vi "ComputeROIArray.vi"(7 "ROIDim":T1, 8 "error in (no error)":errorcluster, 10 "ROI In":T2 {"Contours"."Type" items=["No Selection", "Point", "Line", "Rectangle", "Oval", "Polygon", "Freehand Region", "Annulus", "Unused2", "Unused3", "Broken Line", "Freehand Line", "Rotated Rectangle"]}) -> (0 "error out":errorcluster, 2 "ROIs Out":T2[](array[typedef]) {"Contours"."Type" items=["No Selection", "Point", "Line", "Rectangle", "Oval", "Polygon", "Freehand Region", "Annulus", "Unused2", "Unused3", "Broken Line", "Freehand Line", "Rotated Rectangle"]})   [LabVIEW 2019]
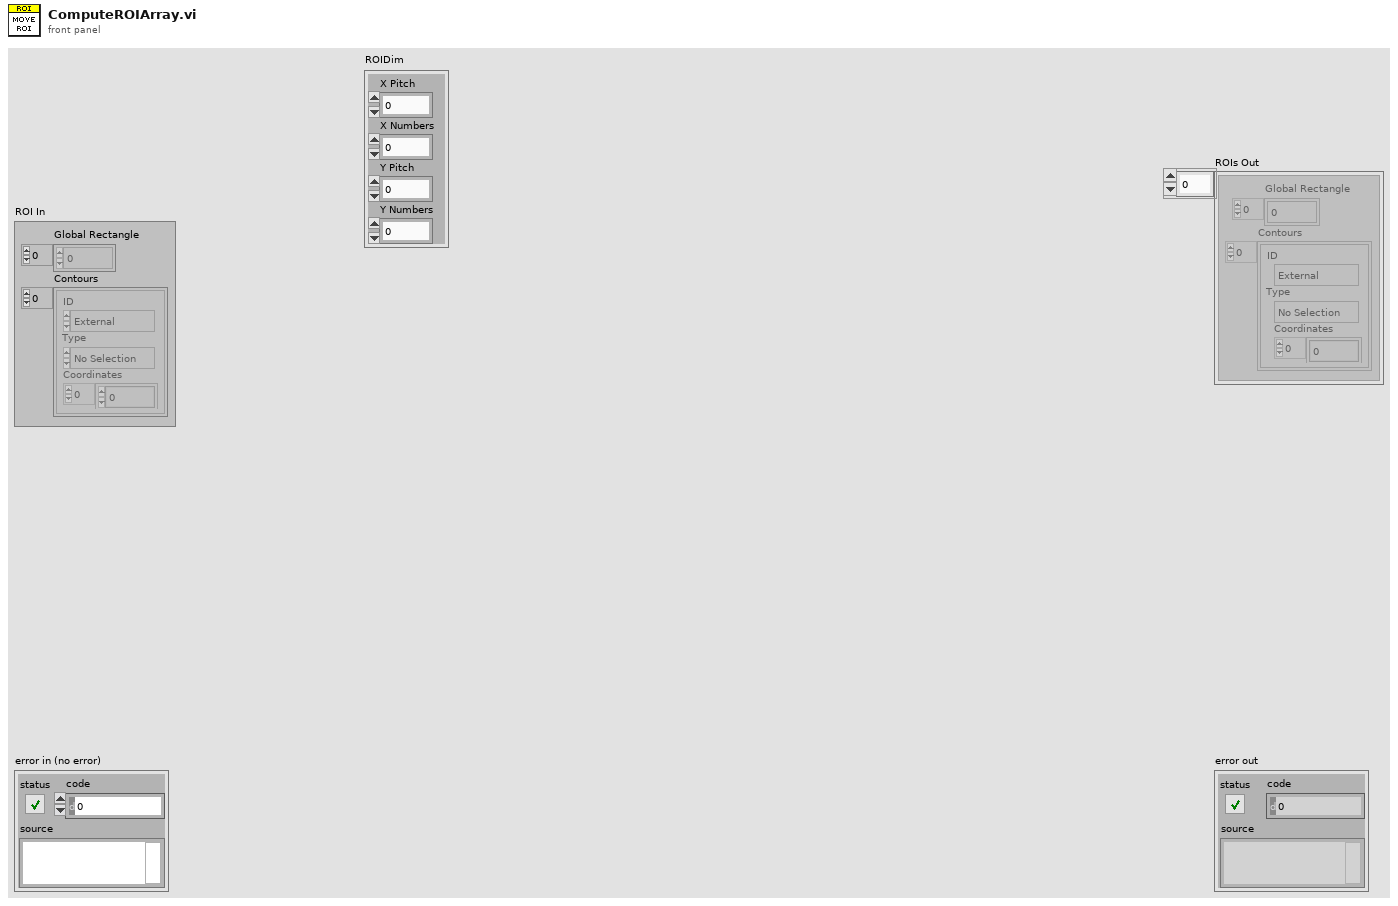
[diagram p1: front panel]
types:
  T1 = cluster{"X Pitch":i32, "X Numbers":i32, "Y Pitch":i32, "Y Numbers":i32}
  T2 = typedef "ROI Descriptor" = cluster{"Global Rectangle":i32[], "Contours":cluster{"ID":enum32{"External", "Internal"}, "Type":u32, "Coordinates":i32[]}[]}
  T3 = cluster{"ID":enum32{"External", "Internal"}, "Type":u32, "Coordinates":i32[]}[]
  T4 = cluster{"ID":enum32{"External", "Internal"}, "Type":u32, "Coordinates":i32[]}
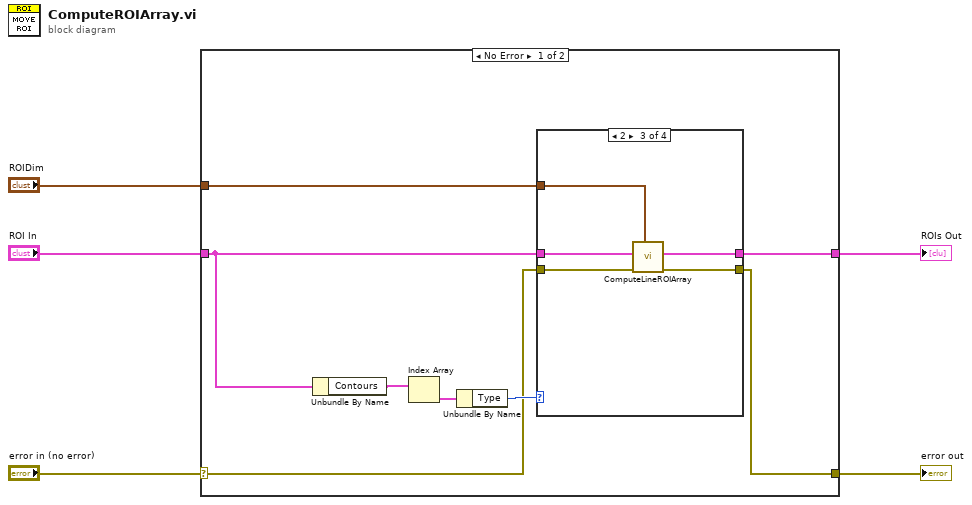
[diagram p0: block diagram]
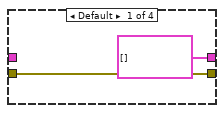
[diagram p2: hidden frame]
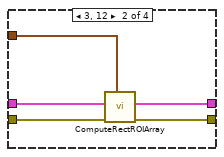
[diagram p3: hidden frame]
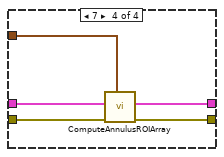
[diagram p4: hidden frame]
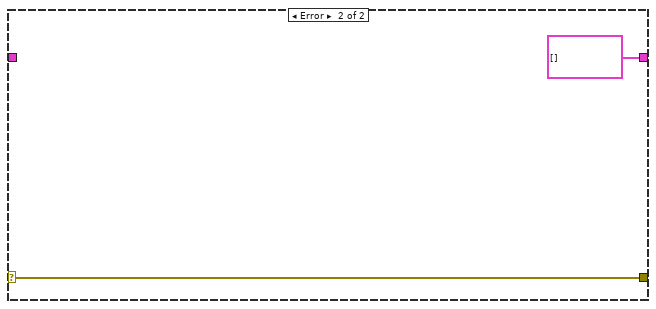
[diagram p5: hidden frame]
diagram:
  n1 = case shown="No Error" "error in (no error)" {
    selector: "error in (no error)" -> [w9 w32]
    tunnel: "ROI In" -> [w13 _]
    tunnel: [w8 w32] -> w3
    tunnel: [w7 T2[] [] ("ROIArray")] -> w2
    tunnel: "ROIDim" -> [w6 _]
    frame No Error {
      n2 = Unbundle By Name(w13) -> ("Contours"=w12:T3)
      n3 = Index Array(array=w12) -> (element=w11:T4)  [unwired: 1 in]
      n4 = Unbundle By Name(w11) -> ("Type"=w10:u32)
      n5 = case shown="2" w10 {
        tunnel: [T2[] [] ("ROIArray") w20 w25 w30] -> w7
        tunnel: [w15 w19 w24 w29] -> w8
        tunnel: w13 -> [_ w18 w22 w28]
        tunnel: w9 -> [w15 w17 w23 w27]
        tunnel: w6 -> [_ w16 w21 w26]
        frame Default {
        }
        frame 3, 12 {
          n6 = call "ComputeRectROIArray.vi"("ROIDim"=w16, "error in (no error)"=w17, "ROI In"=w18) -> ("error out"=w19:errorcluster, "ROIArray"=w20:T2[])  [unwired: 7 in]
        }
        frame 2 {
          n7 = call "ComputeLineROIArray.vi"("ROIDim"=w21, "error in (no error)"=w23, "ROI In"=w22) -> ("error out"=w24:errorcluster, "ROIArray"=w25:T2[])  [unwired: 7 in]
        }
        frame 7 {
          n8 = call "ComputeAnnulusROIArray.vi"("ROIDim"=w26, "error in (no error)"=w27, "ROI In"=w28) -> ("error out"=w29:errorcluster, "ROIArray"=w30:T2[])  [unwired: 7 in]
        }
      }
    }
    frame Error {
    }
  }
  "error out" <- w3
  "ROIs Out" <- w2
